vi "Create Test Classes.vi"(4 "error in":errorcluster) -> (0 "error out":errorcluster)   [LabVIEW 2025]
doc: "This VI creates all configured test classes for unit testing. The configuration file <i>Test Class Definition.xml</i> must lie in the same folder as this VI."
uses:
  Class Definition--cluster.ctl
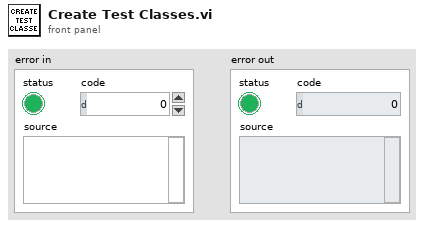
[diagram p1: front panel]
types:
  T1 = typedef "Class Definition--cluster.ctl" = cluster{"Name":string, "Description":string}
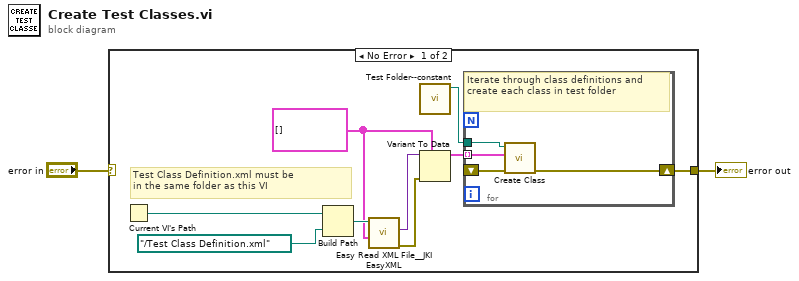
[diagram p0: block diagram]
diagram:
  n1 = case shown="No Error" "error in" {
    selector: "error in" -> [_ w16]
    tunnel: [w9 w16] -> w1
    frame No Error {
      w3 = T1[] [] ("Array")
      # "Test Class Definition.xml must be\nin the same folder as this VI"
      n2 = Current VI's Path() -> (path=w11:path)
      n3 = Build Path(base path=w11, name or relative path=path "../Test Class Definition.xml") -> (appended path=w6:path)
      n4 = call <vilib>:"Easy Read XML File__JKI EasyXML.vi"("LabVIEW Data (Type)"=w3, "XML File Path"=w6) -> ("error out"=w5:errorcluster, "LabVIEW Data"=w4:variant)  [unwired: 7 in, 1 out]
      n5 = call "Test Folder--constant.vi"() -> ("Test Folder"=w8:path)  [unwired: 7 in]
      n6 = Variant To Data(error in=w5, type=w3, Variant=w4) -> (data=w7:T1[])  [unwired: 1 out]
      n7 = for {
        tunnel: w8 -> [w15]
        tunnel: w7 -> [w14] mode=indexing
        shift-right: [w12] -> w9
        shift-left: _ -> [w13]
        # "Iterate through class definitions and create each class in test folder"
        n8 = call "Create Class.vi"("error in"=w13, "Class Definition"=w14, "Path"=w15) -> ("error out"=w12:errorcluster)  [unwired: 4 in]
      }
    }
    frame Error {
      # "Pass error without further action"
    }
  }
  "error out" <- w1
